vi "Respond Box.vi"(5 "error in":errorcluster, 6 "Play?":bool=TRUE, 7 "Trial#":u16, 8 "target":dbl) -> (0 "Force":dbl[](array[numeric]), 1 "out":i8, 2 "Correct?":bool)   [LabVIEW 2012]
uses:
  Global_var.vi
  <userlib>/dhd_sdk7/dhd_sdk7.lvlib
panel:
  out "Boolean":bool
  out "Respond":string
  out "error out":errorcluster
  out "Correct \nAnswer":string
  in  "RefAnswer":u8[](array[numeric])
  in  "2":bool
  in  "1":bool
  # "Trial number:"
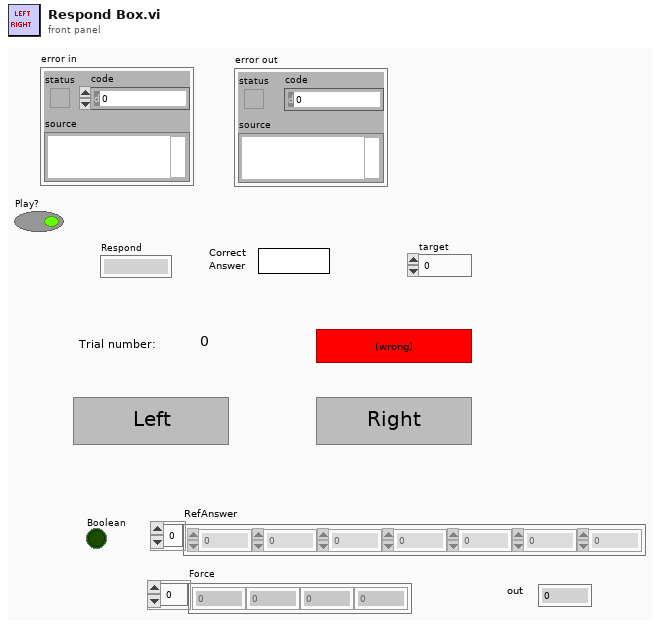
[diagram p1: front panel]
types:
  T1 = typedef "Sound Output Task ID.ctl" = u32
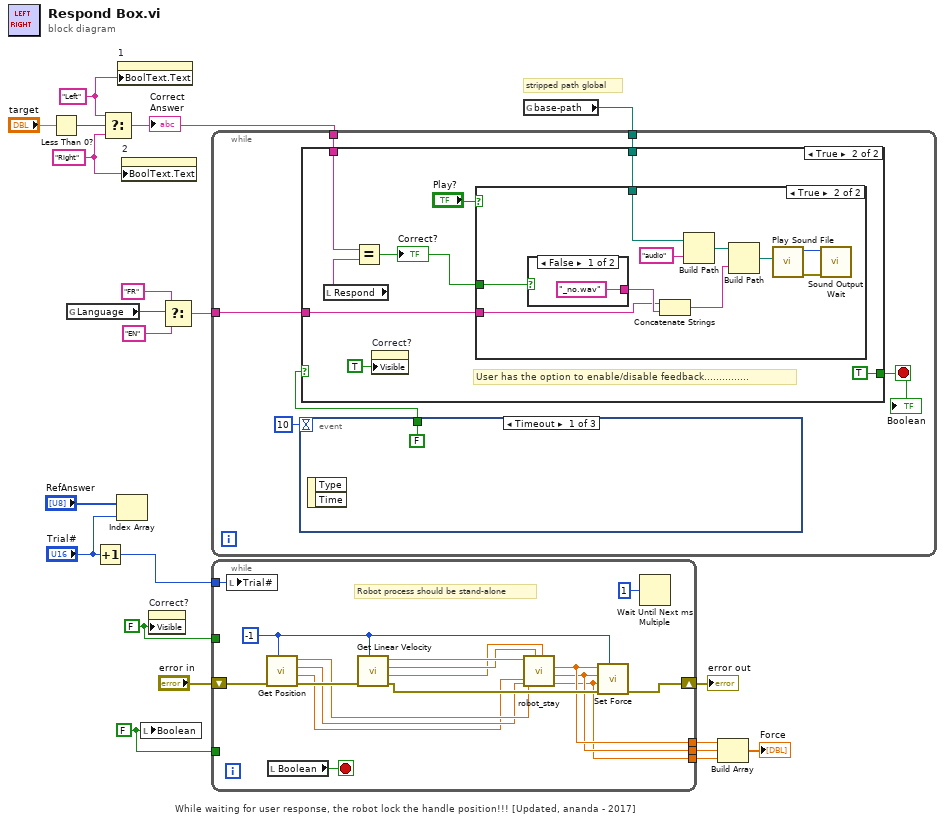
[diagram p0: block diagram]
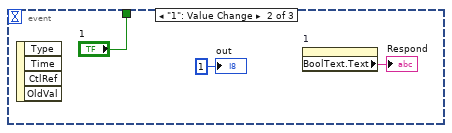
[diagram p2: hidden frame]
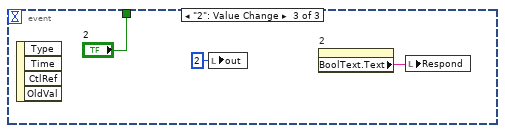
[diagram p3: hidden frame]
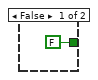
[diagram p4: hidden frame]
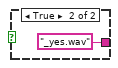
[diagram p6: hidden frame]
diagram:
  w1 = FALSE ("Boolean")
  w8 = FALSE ("Visible")
  w15 = "Right" ("Correct Answer")
  w19 = "Left" ("Correct Answer")
  # "stripped path global"
  # "While waiting for user response, the robot lock the handle position!!! [Updated, ananda - 2017]"
  n1 = Less Than 0?(x="target") -> (x < 0?=w14:bool)
  n2 = global read "Global_var.vi" "Language"() -> (w6:bool)
  n3 = Increment(x="Trial#") -> (x+1=w2:u16)
  n4 = Select(t=w19, s=w14, f=w15) -> (s? t:f=w20:string)
  "Correct \nAnswer" <- w20
  n5 = Index Array(array="RefAnswer", index="Trial#") -> ()  [unwired: 1 out]
  n6 = property on="1" class="Bool"("BoolText.Text"=w19) -> ()  [unwired: 2 in, 2 out]
  n7 = property on="2" class="Bool"("BoolText.Text"=w15) -> ()  [unwired: 2 in, 2 out]
  n8 = local write "Boolean"(w1) -> ()
  n9 = property on="Correct?" class="Bool (strict)"("Visible"=w8) -> ()  [unwired: 2 in, 2 out]
  n10 = Select(t="FR" ("Correct Answer"), s=w6, f="EN" ("Correct Answer")) -> (s? t:f=w3:string)
  n11 = while {
    shift-right: [w34] -> w17
    shift-left: "error in" -> [w38]
    tunnel: [w27] -> w11
    tunnel: [w26] -> w10
    tunnel: [w25] -> w9
    tunnel: w8 -> [_]
    tunnel: w2 -> [w23]
    tunnel: w1 -> [_]
    stop <- w24 stop-if-true
    w35 = i8 -1 ("ID")
    # "Robot process should be stand-alone"
    n12 = local write "Trial#"(w23) -> ()
    n13 = call <userlib>:"Get Position.vi"("ID"=w35, "error in (no error)"=w38) -> ("error out"=w37:errorcluster, "pz out"=w28:dbl, "py out"=w29:dbl, "px out"=w30:dbl)  [unwired: 5 in, 1 out]
    n14 = local read "Boolean"() -> (w24:bool)
    n15 = call <userlib>:"Get Linear Velocity.vi"("ID"=w35, "error in (no error)"=w37) -> ("error out"=w36:errorcluster, "vz out"=w31:dbl, "vy out"=w32:dbl, "vx out"=w33:dbl)  [unwired: 5 in, 1 out]
    n16 = call "robot_stay.vi"("Vz"=w31, "Z"=w28, "Vy"=w32, "Y"=w29, "X"=w30, "Vx"=w33) -> ("Fz"=w25:dbl, "Fy"=w26:dbl, "Fx"=w27:dbl)  [unwired: 3 in]
    n17 = call <userlib>:"Set Force.vi"("ID"=w35, "error in (no error)"=w36, "fz"=w25, "fy"=w26, "fx"=w27) -> ("error out"=w34:errorcluster)  [unwired: 5 in, 1 out]
    n18 = Wait Until Next ms Multiple(millisecond multiple=u32 1) -> ()  [unwired: 1 out]
  }
  "error out" <- w17
  n19 = global read "Global_var.vi" "base-path"() -> (w7:path)
  n20 = while {
    tunnel: w20 -> [w44]
    tunnel: w7 -> [w43]
    tunnel: w3 -> [w41]
    stop <- w42 stop-if-true
    n21 = event shown="[0] Timeout" {
      selector: _ -> [_ _ _]
      dyn-events: _ -> [_ _ _]
      timeout: 10 -> [_ _ _]
      tunnel: [FALSE ("2") "1" "2"] -> w39
      event Timeout {
        n22 = event-data() -> ()  [unwired: 1 in, 2 out]
      }
      event "1": Value Change {
        n23 = event-data() -> ()  [unwired: 1 in, 4 out]
        n24 = property on="1" class="Bool"() -> ("BoolText.Text"=→"Respond":string)  [unwired: 2 in, 2 out]
        "out" <- i8 1 ("millisecond multiple")
      }
      event "2": Value Change {
        n25 = event-data() -> ()  [unwired: 1 in, 4 out]
        n26 = local write "out"(i8 2 ("millisecond multiple")) -> ()
        n27 = property on="2" class="Bool"() -> ("BoolText.Text"=w50:string)  [unwired: 2 in, 2 out]
        n28 = local write "Respond"(w50) -> ()
      }
    }
    n29 = case shown="True" w39 {
      tunnel: w44 -> [_ w59]
      tunnel: w43 -> [_ w58]
      tunnel: [FALSE TRUE] -> w42
      tunnel: w41 -> [_ w53]
      frame False {
      }
      frame True {
        # "User has the option to enable/disable feedback..............."
        n30 = local read "Respond"() -> (w54:string)
        n31 = Equal?(x=w59, y=w54) -> (x = y?=w60:bool)
        "Correct?" <- w60
        n32 = property on="Correct?" class="Bool (strict)"("Visible"=TRUE) -> ()  [unwired: 2 in, 2 out]
        n33 = case shown="True" "Play?" {
          tunnel: w58 -> [_ w66]
          tunnel: w60 -> [_ w64]
          tunnel: w53 -> [_ w61]
          frame False {
            # "Play only durimg training!!\nFor \"Test extreme\", it is off!"
          }
          frame True {
            n34 = case shown="False" w64 {
              tunnel: ["_no.wav" ("name or relative path") "_yes.wav" ("name or relative path")] -> w63
              frame False {
              }
              frame True {
              }
            }
            n35 = Concatenate Strings(w61, w63) -> (w62:string)
            n36 = Build Path(base path=w66, name or relative path="audio") -> (appended path=w68:path)
            n37 = Build Path(base path=w68, name or relative path=w62) -> (appended path=w65:path)
            n38 = call <vilib>:"Play Sound File.vi"("path"=w65) -> ("error out"=w70:errorcluster, "task ID"=w69:T1)  [unwired: 9 in]
            n39 = call <vilib>:"Sound Output Wait.vi"("error in (no error)"=w70, "task ID"=w69) -> ()  [unwired: 8 in, 2 out]
          }
        }
      }
    }
    "Boolean" <- w42
  }
  n40 = Build Array(w11, w10, w9) -> (→"Force":dbl[])
